vi "Re-Sort SubComponents.vi"(8 "error in (no error)":errorcluster, 11 "1553 Component in":refnum<class "1553 Component.lvclass">) -> (0 "error out":errorcluster, 3 "1553 Component out":refnum<class "1553 Component.lvclass">)   [LabVIEW 2016, in "BCI-1553 API.lvlib" / "1553 Component.lvclass"]
doc: "Requests each of the SubComponents this Component ihas to resort themselves into a know and ideal order for memory utilization."
uses:
  1553 Component.lvclass
  1553 SubComponent/1553 SubComponent.lvclass
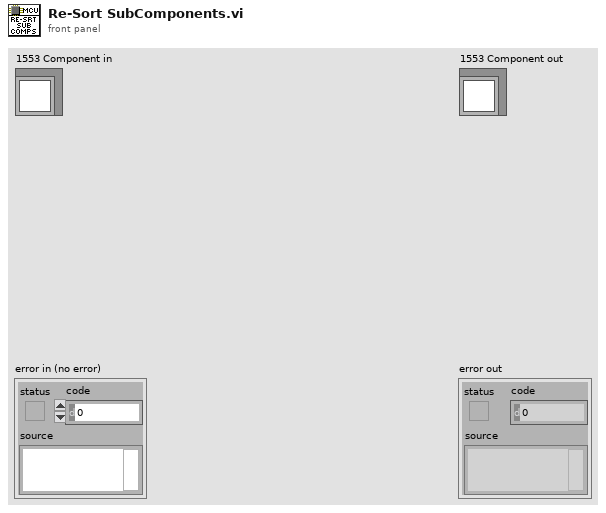
[diagram p1: front panel]
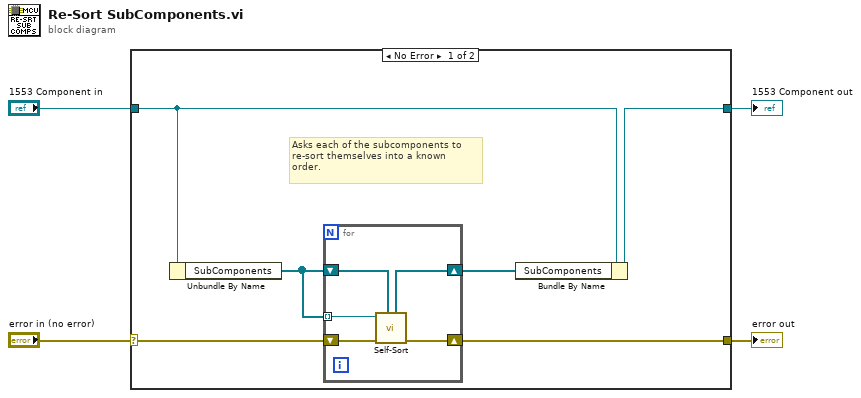
[diagram p0: block diagram]
diagram:
  n1 = case shown="No Error" "error in (no error)" {
    selector: "error in (no error)" -> [w8 w17]
    tunnel: [w7 w17] -> w3
    tunnel: [w9 w16] -> w1
    tunnel: "1553 Component in" -> [w10 w16]
    frame No Error {
      # "Asks each of the subcomponents to\nre-sort themselves into a known\norder."
      n2 = Unbundle By Name(w10) -> ("SubComponents"=w5:refnum<class "1553 SubComponent.lvclass">[])
      n3 = for {
        shift-right: [w14] -> w7
        shift-left: w8 -> [w15]
        shift-right: [w13] -> w6
        shift-left: w5 -> [w12]
        tunnel: w5 -> [w11] mode=indexing
        n4 = call-dynamic "Self-Sort.vi"("SubComponent List"=w12, "error in (no error)"=w15, "1553 SubComponent in"=w11) -> ("error out"=w14:errorcluster, "SubComponent List out"=w13:refnum<class "1553 SubComponent.lvclass">[])  [unwired: 7 in]
      }
      n5 = Bundle By Name(cluster=w10, "SubComponents"=w6) -> (w9:refnum<class "1553 Component.lvclass">)
    }
    frame Error {
    }
  }
  "error out" <- w3
  "1553 Component out" <- w1
